vi "AddNewConnection.vi"(3 "error in (no error)":errorcluster, 5 "data":T1={"New Subscriber"={"Caller ID"="", "Topic Name"="", "Protocol"="", "URIs"="", "ID"=refnum}, "ROS of Server"={"topic port"=0, "Node"="", "topic"="", "type"="", "node port"=0, "error "={"status"=FALSE, "code"=0, "source"=""}, "Direction"=enum."Node", "APIs"=[], "Update (ms)"=1, "write queue"=1}, "new port"=0}) -> (0 "error out":errorcluster)   [LabVIEW 2010]
uses:
  SubVIs/_ROSDirection.ctl
  SubVIs/_ROSControl.ctl
  requestTopic.ctl
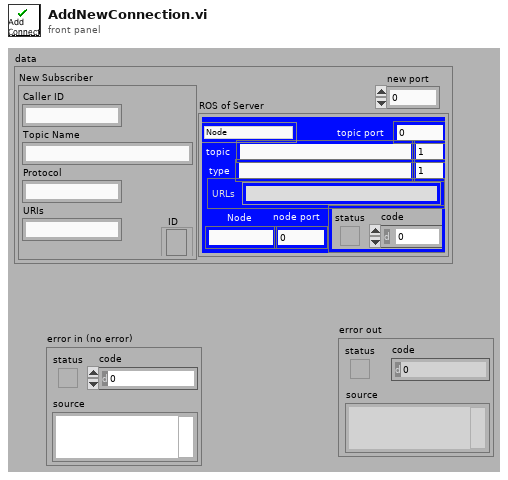
[diagram p1: front panel]
types:
  T1 = typedef "requestTopic.ctl" = cluster{"New Subscriber":cluster{"Caller ID":string, "Topic Name":string, "Protocol":string, "URIs":string, "ID":refnum<k5>}, "ROS of Server":T2, "new port":u16}
  T2 = typedef "_ROSControl.ctl" = cluster{"topic port":u16, "Node":string, "topic":string, "type":string, "node port":u32, "error ":errorcluster, "Direction":T3, "APIs":string[], "Update (ms)":u16, "write queue":u16}
  T3 = typedef "_ROSDirection.ctl" = enum16{"Node", "Publisher", "Subscriber", "Service Client"}
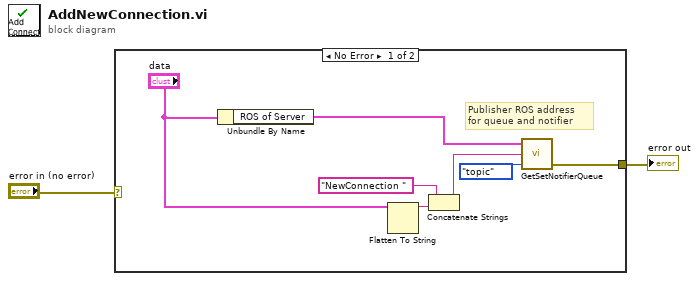
[diagram p0: block diagram]
diagram:
  n1 = case shown="No Error" "error in (no error)" {
    selector: "error in (no error)" -> [_ w10]
    tunnel: [w4 w10] -> w1
    frame No Error {
      # "Publisher ROS address \nfor queue and notifier"
      n2 = Unbundle By Name("data") -> ("ROS of Server"=w3:T2)
      n3 = Flatten To String(anything="data") -> (data string=w7:string)  [unwired: 3 in, 2 out]
      n4 = Concatenate Strings("NewConnection " ("Command"), w7) -> (w5:string)
      n5 = call "GetSetNotifierQueue.vi"("Name"=enum16{"topic", "node"}."topic", "Command"=w5, "ROS"=w3) -> ("error out"=w4:errorcluster)  [unwired: 2 out]
    }
    frame Error {
    }
  }
  "error out" <- w1
